vi "create_mission_waypoints.vi"(9 "Mission in":refnum<class "Mission.lvclass">) -> (1 "Mission out":refnum<class "Mission.lvclass">)   [LabVIEW 2011, in "Mission.lvclass"]
uses:
  Mission.lvclass
  Mission.lvclass/Mission.ctl
  2 Globals/2 Global.vi
  Waypoint/Waypoint.lvclass
panel:
  in  "Tolerance":dbl
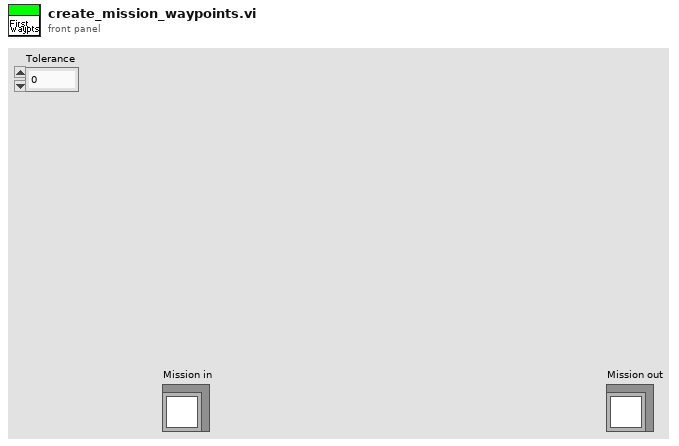
[diagram p1: front panel]
types:
  T1 = enum16{"Round Buoy", "Drive", "Pass Buoys", "Station Keeping"}
  T2 = typedef "UTM Location.ctl" = cluster{"UTM Zone":dbl, "Hemisphere":enum16{"North", "South"}, "East":dbl, "North":dbl}
  T3 = typedef "Waypoints List.ctl" = refnum<class "Waypoint.lvclass">[]
  T4 = typedef "UTM Circle.ctl" = cluster{"UTM Zone":dbl, "Hemisphere":enum16{"North", "South"}, "East":dbl, "North":dbl, "Radius":dbl}
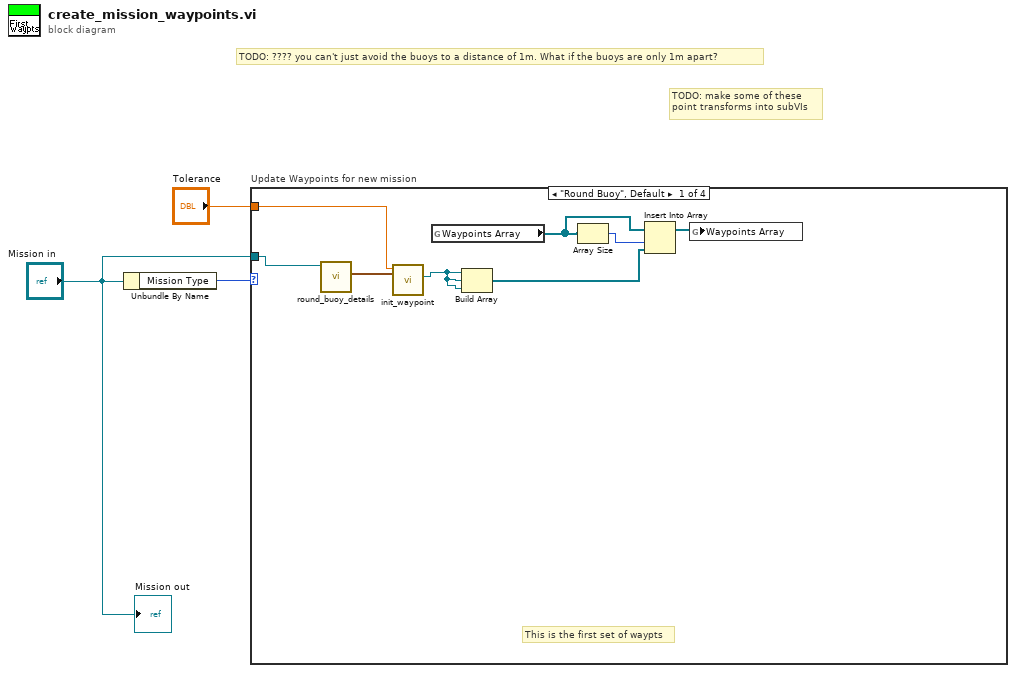
[diagram p0: block diagram]
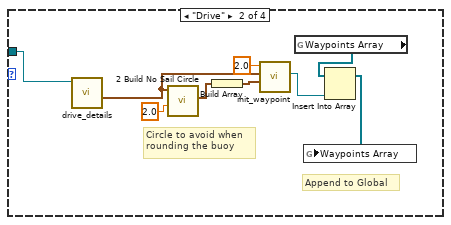
[diagram p2: hidden frame]
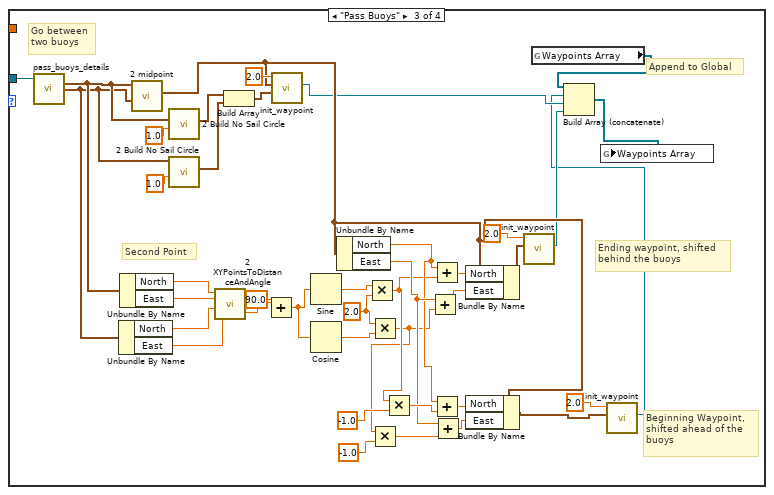
[diagram p3: hidden frame]
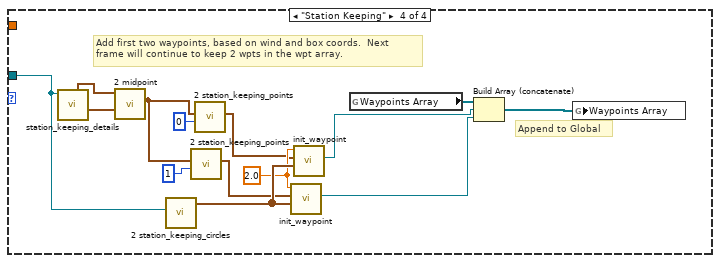
[diagram p4: hidden frame]
diagram:
  # "TODO: make some of these\npoint transforms into subVIs"
  # "TODO: ???? you can't just avoid the buoys to a distance of 1m. What if the buoys are only 1m apart?"
  n1 = Unbundle By Name("Mission in") -> ("Mission Type"=w3:T1)
  n2 = case "Update Waypoints for new mission" shown="\"Round Buoy\", Default" w3 {
    tunnel: "Mission in" -> [w11 w14 w57 w70]
    tunnel: "Tolerance" -> [w9 _ _ _]
    frame "Round Buoy", Default {
      # "This is the first set of waypts"
      n3 = call-dynamic "round_buoy_details.vi"("Mission in"=w11) -> ("Buoy to Round"=w10:T2)  [unwired: 7 in, 3 out]
      n4 = call "init_waypoint.vi"("Coords"=w10, "Tolerance (m)"=w9) -> ("Waypoint Out"=w8:refnum<class "Waypoint.lvclass">)  [unwired: 9 in]
      n5 = global read "2 Global.vi" "Waypoints Array"() -> (w6:T3)
      n6 = Build Array(w8, w8, w8) -> (w5:refnum<class "Waypoint.lvclass">[])
      n7 = Array Size(array=w6) -> (size(s)=w7:i32)
      n8 = Insert Into Array(array=w6, index=w7, new element=w5) -> (w4:T3)
      n9 = global write "2 Global.vi" "Waypoints Array"(w4) -> ()
    }
    frame "Drive" {
      # "Append to Global"
      # "Circle to avoid when\nrounding the buoy"
      n10 = call-dynamic "drive_details.vi"("Mission in"=w14) -> ("Drive Location"=w13:T2)  [unwired: 8 in, 2 out]
      n11 = call "2 Build No Sail Circle.vi"("Radius"=2.0, "UTM Location"=w13) -> ("UTM Circle"=w19:T4)  [unwired: 9 in]
      n12 = Build Array(w19) -> (w20:T4[])
      n13 = call "init_waypoint.vi"("No Sail Circles"=w20, "Coords"=w13, "Tolerance (m)"=2.0 ("Tolerance (meters?)")) -> ("Waypoint Out"=w12:refnum<class "Waypoint.lvclass">)  [unwired: 8 in]
      n14 = global read "2 Global.vi" "Waypoints Array"() -> (w15:T3)
      n15 = Insert Into Array(array=w15, new element=w12) -> (w16:T3)  [unwired: 1 in]
      n16 = global write "2 Global.vi" "Waypoints Array"(w16) -> ()
    }
    frame "Pass Buoys" {
      w37 = 2.0 ("Tolerance (meters?)")
      # "Ending waypoint, shifted\nbehind the buoys"
      # "Beginning Waypoint,\nshifted ahead of the\nbuoys"
      # "Second Point"
      # "Go between\ntwo buoys"
      # "Append to Global"
      n17 = call-dynamic "pass_buoys_details.vi"("Mission in"=w57) -> ("Buoy Pass Port"=w52:T2, "Buoy Pass Starboard"=w51:T2)  [unwired: 11 in, 2 out]
      n18 = Unbundle By Name(w51) -> ("North"=w48:dbl, "East"=w47:dbl)
      n19 = Unbundle By Name(w52) -> ("North"=w50:dbl, "East"=w49:dbl)
      n20 = call "2 midpoint.vi"("UTM 2"=w51, "UTM 1"=w52) -> ("Midpoint"=w26:T2)  [unwired: 8 in, 1 out]
      n21 = call "2 Build No Sail Circle.vi"("Radius"=1.0, "UTM Location"=w52) -> ("UTM Circle"=w60:T4)  [unwired: 9 in]
      n22 = call "2 Build No Sail Circle.vi"("Radius"=1.0, "UTM Location"=w51) -> ("UTM Circle"=w56:T4)  [unwired: 9 in]
      n23 = call "2 XYPointsToDistanceAndAngle.vi"("East 2"=w47, "North 2"=w48, "East 1"=w49, "North 1"=w50) -> ("Angle Diff"=w46:dbl)  [unwired: 1 out]
      n24 = Build Array(w60, w56) -> (w61:T4[])
      n25 = Add(x=w46, y=90.0 ("Radius")) -> (x+y=w44:dbl)
      n26 = call "init_waypoint.vi"("No Sail Circles"=w61, "Coords"=w26, "Tolerance (m)"=2.0 ("Tolerance (meters?)")) -> ("Waypoint Out"=w22:refnum<class "Waypoint.lvclass">)  [unwired: 8 in]
      n27 = Sine(x=w44) -> (sin(x)=w39:dbl)
      n28 = Cosine(x=w44) -> (cos(x)=w38:dbl)
      n29 = Unbundle By Name(w26) -> ("North"=w31:dbl, "East"=w32:dbl)
      n30 = Multiply(x=w39, y=w37) -> (x*y=w30:dbl)
      n31 = Multiply(x=w37, y=w38) -> (x*y=w29:dbl)
      n32 = Multiply(x=w29, y=-1.0 ("Tolerance (meters?)")) -> (x*y=w34:dbl)
      n33 = Multiply(x=w30, y=-1.0 ("Tolerance (meters?)")) -> (x*y=w33:dbl)
      n34 = Add(x=w32, y=w29) -> (x+y=w43:dbl)
      n35 = Add(x=w31, y=w30) -> (x+y=w42:dbl)
      n36 = Add(x=w31, y=w33) -> (x+y=w28:dbl)
      n37 = Add(x=w32, y=w34) -> (x+y=w27:dbl)
      n38 = Bundle By Name(cluster=w26, "North"=w42, "East"=w43) -> (w41:T2)
      n39 = Bundle By Name(cluster=w26, "North"=w28, "East"=w27) -> (w24:T2)
      n40 = call "init_waypoint.vi"("Coords"=w41, "Tolerance (m)"=2.0 ("Tolerance (meters?)")) -> ("Waypoint Out"=w23:refnum<class "Waypoint.lvclass">)  [unwired: 9 in]
      n41 = global read "2 Global.vi" "Waypoints Array"() -> (w54:T3)
      n42 = call "init_waypoint.vi"("Coords"=w24, "Tolerance (m)"=2.0 ("Tolerance (meters?)")) -> ("Waypoint Out"=w21:refnum<class "Waypoint.lvclass">)  [unwired: 9 in]
      n43 = Build Array (concatenate)(w54, w21, w22, w23) -> (w53:T3)
      n44 = global write "2 Global.vi" "Waypoints Array"(w53) -> ()
    }
    frame "Station Keeping" {
      w68 = 2.0 ("Tolerance (meters?)")
      # "Append to Global"
      # "Add first two waypoints, based on wind and box coords.  Next\nframe will continue to keep 2 wpts in the wpt array."
      n45 = call-dynamic "station_keeping_details.vi"("Mission in"=w70) -> ("Buoy SE"=w74:T2, "Buoy NW"=w75:T2)  [unwired: 4 in, 5 out]
      n46 = call "2 midpoint.vi"("UTM 2"=w74, "UTM 1"=w75) -> ("Midpoint"=w65:T2)  [unwired: 8 in, 1 out]
      n47 = call "2 station_keeping_circles.vi"("Mission in"=w70) -> ("No Sail Circles"=w69:T4[])  [unwired: 10 in]
      n48 = call "2 station_keeping_points.vi"("Which Point?"=1, "Midpoint"=w65) -> ("Waypoint"=w67:T2)  [unwired: 9 in]
      n49 = call "2 station_keeping_points.vi"("Which Point?"=0, "Midpoint"=w65) -> ("Waypoint"=w66:T2)  [unwired: 9 in]
      n50 = call "init_waypoint.vi"("No Sail Circles"=w69, "Coords"=w67, "Tolerance (m)"=w68) -> ("Waypoint Out"=w71:refnum<class "Waypoint.lvclass">)  [unwired: 8 in]
      n51 = call "init_waypoint.vi"("No Sail Circles"=w69, "Coords"=w66, "Tolerance (m)"=w68) -> ("Waypoint Out"=w72:refnum<class "Waypoint.lvclass">)  [unwired: 8 in]
      n52 = global read "2 Global.vi" "Waypoints Array"() -> (w73:T3)
      n53 = Build Array (concatenate)(w73, w72, w71) -> (w62:T3)
      n54 = global write "2 Global.vi" "Waypoints Array"(w62) -> ()
    }
  }
  "Mission out" <- "Mission in"
